vi "UPTEST.vi"(6 "错误输入":errorcluster, 7 "Result":string[][](table), 8 "CODE_ID":string, 9 "DEVICE_ID":string) -> (0 "错误输出":errorcluster caption="错误输入")   [LabVIEW 2020]
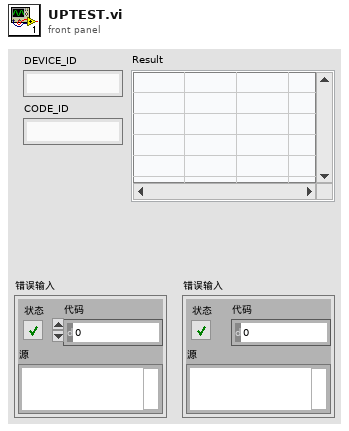
[diagram p1: front panel]
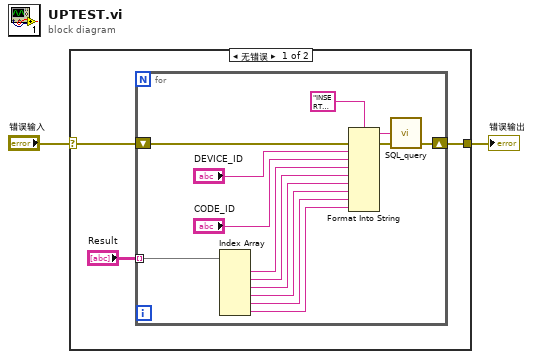
[diagram p0: block diagram]
diagram:
  n1 = case shown="无错误" "错误输入" {
    selector: "错误输入" -> [w3 w20]
    tunnel: [w4 w20] -> w1
    frame No Error {
      n2 = for {
        tunnel: "Result" -> [w19] mode=indexing
        shift-right: [w11] -> w4
        shift-left: w3 -> [w10]
        n3 = Index Array(array=w19) -> (element #1=w18:string, element #2=w17:string, element #3=w16:string, element #4=w15:string, element #5=w14:string, element #6=w7:string)  [unwired: 6 in]
        n4 = Format Into String(format string="INSERT INTO [dbo].[Test] ( [DEVICE_ID], [CODE_ID], [TEST_NAME], [TEST_VALUE], [TEST_VALUE_MIN], [TEST_VALUE_MAX], [TEST_VALUE_UNIT], [TEST_VALUE_RESULT] )\nVALUES\n\t( %s, %s, N'%s', %s, %s, %s, '%s', '%s' )", error in=w10, "DEVICE_ID", "CODE_ID", w18, w17, w16, w15, w14, w7) -> (resulting string=w13:string, error out=w12:errorcluster)  [unwired: 1 in]
        n5 = call "SQL_query.vi"("error in (no error)"=w12, "SQL query"=w13) -> ("error out"=w11:errorcluster)  [unwired: 2 in, 1 out]
      }
    }
    frame Error {
    }
  }
  "错误输出" <- w1
